vi "MVE Help.vi"   [LabVIEW 2016]
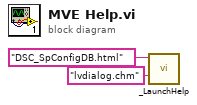
[diagram p0: block diagram]
diagram:
  n1 = call <helpdir>:"_LaunchHelp.vi"("CHM or HLP filename (lvdialog.chm)"="lvdialog.chm", "HTML filename"="DSC_SpConfigDB.html") -> ()  [unwired: 5 in, 1 out]
